vi "Normalize Image.vi"(8 "error in (no error)":errorcluster, 11 "Image In":T1) -> (0 "error out":errorcluster, 3 "Image Out":T1)   [LabVIEW 2016]
uses:
  <vilib>/vision/Image Controls.llb/IMAQ Image.ctl
  <vilib>/vision/NI_Vision_Development_Module.lvlib
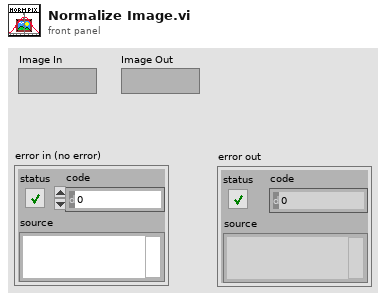
[diagram p1: front panel]
types:
  T1 = typedef "IMAQ Image.ctl" = refnum<image>
  T2 = cluster{"histogram":u32[], "Minimal Value":sgl, "Maximal Value":sgl, "Starting Value":sgl, "Interval Width":sgl, "Mean Value":sgl, "Standard  Variation":sgl, "Area (pixels)":i32}
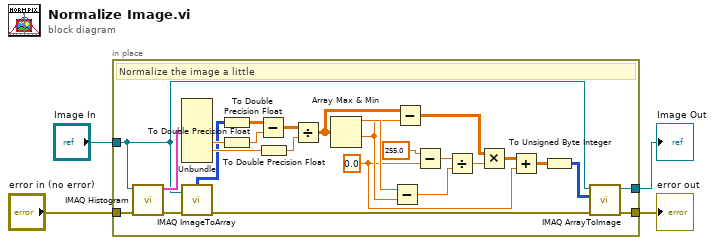
[diagram p0: block diagram]
diagram:
  n1 = in-place {
    in-place-border: "Image In" -> [w13]
    in-place-border: [w14] -> w3
    in-place-border: "error in (no error)" -> [w8]
    in-place-border: [w5] -> w1
    w15 = 0.0
    # "Normalize the image a little"
    n2 = call "IMAQ Histogram"("error in (no error)"=w8, "Image"=w13) -> ("error out"=w7:errorcluster, "Histogram Report"=w30:T2)  [unwired: 8 in]
    n3 = Unbundle(w30) -> ("Mean Value"=w29:sgl, "Standard  Variation"=w27:sgl)  [unwired: 6 out]
    n4 = call "IMAQ ImageToArray"("error in (no error)"=w7, "Image"=w13) -> ("error out"=w6:errorcluster, "Image Pixels (U8)"=w9:u8[][])  [unwired: 2 in, 3 out]
    n5 = To Double Precision Float(number=w9) -> (double precision float=w10:dbl[][])
    n6 = To Double Precision Float(number=w29) -> (double precision float=w26:dbl)
    n7 = Subtract(x=w10, y=w26) -> (x-y=w25:dbl[][])
    n8 = To Double Precision Float(number=w27) -> (double precision float=w24:dbl)
    n9 = Divide(x=w25, y=w24) -> (x/y=w22:dbl[][])
    n10 = Array Max & Min(array=w22) -> (max value=w23:dbl, min value=w21:dbl)  [unwired: 2 out]
    n11 = Subtract(x=w23, y=w21) -> (x-y=w19:dbl)
    n12 = Subtract(x=w22, y=w21) -> (x-y=w18:dbl[][])
    n13 = Subtract(x=255.0, y=w15) -> (x-y=w20:dbl)
    n14 = Divide(x=w20, y=w19) -> (x/y=w17:dbl)
    n15 = Multiply(x=w18, y=w17) -> (x*y=w16:dbl[][])
    n16 = Add(x=w16, y=w15) -> (x+y=w12:dbl[][])
    n17 = To Unsigned Byte Integer(number=w12) -> (unsigned 8bit integer=w11:u8[][])
    n18 = call "IMAQ ArrayToImage"("error in (no error)"=w6, "Image Pixels (U8)"=w11, "Image"=w13) -> ("error out"=w5:errorcluster, "Image Out"=w14:T1)  [unwired: 7 in]
  }
  "Image Out" <- w3
  "error out" <- w1
